vi "perform handshake.vi"(8 "error in":errorcluster, 9 "timeout":i32=-1, 11 "lvlibretls connection in":refnum<class "lvlibretls connection.lvclass">) -> (0 "error out":errorcluster, 3 "lvlibretls connection out":refnum<class "lvlibretls connection.lvclass">)   [LabVIEW 2016, in "lvlibretls connection.lvclass"]
doc: "tls_handshake() explicitly performs the TLS handshake. It is only necessary to call this function if you need to guarantee that the handshake has completed, as both tls_read() and tls_write() automatically perform the TLS handshake when necessary."
uses:
  lvlibretls connection.lvclass
  lvlibretls connection.lvclass/lvlibretls connection.ctl
  tls library paths.vi
  lv tls dll.lvlib
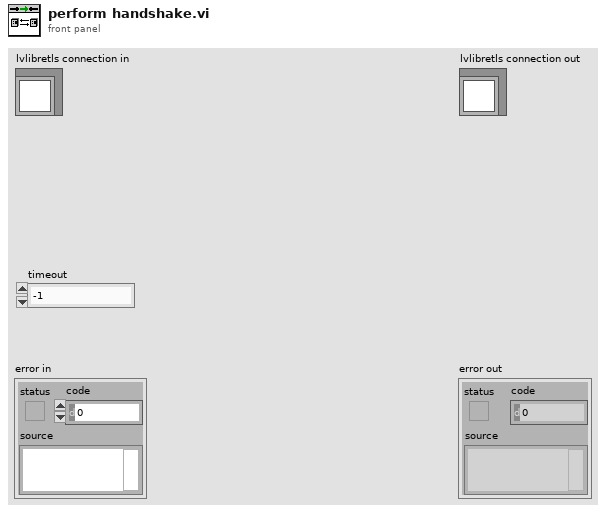
[diagram p1: front panel]
types:
  T1 = enum16{"Standard", "Buffered", "CRLF", "Immediate"}
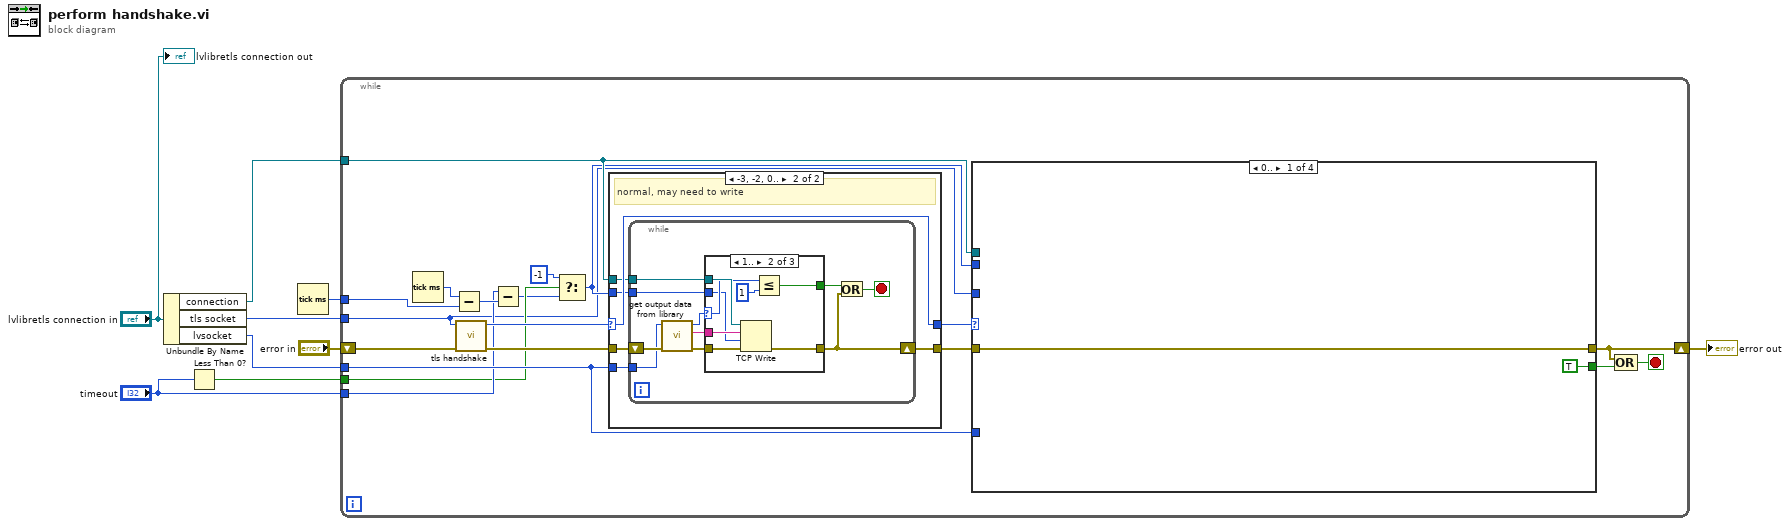
[diagram p0: block diagram]
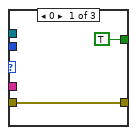
[diagram p3: hidden frame]
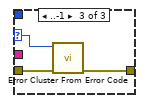
[diagram p4: hidden frame]
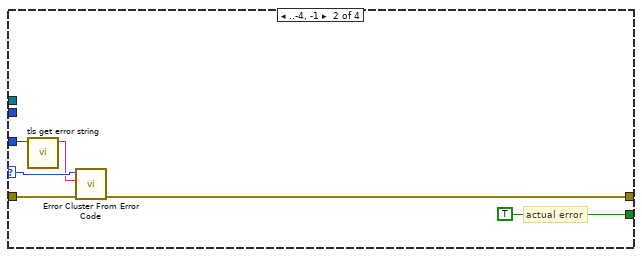
[diagram p5: hidden frame]
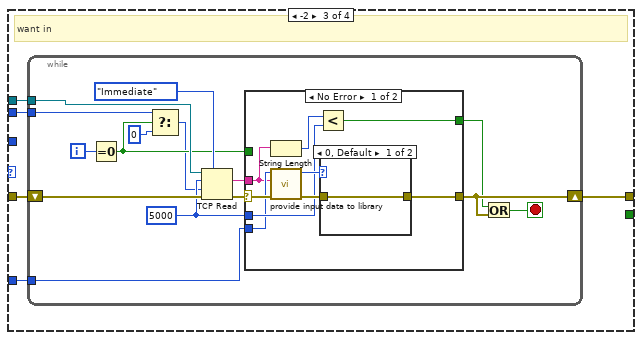
[diagram p6: hidden frame]
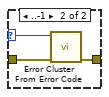
[diagram p7: hidden frame]
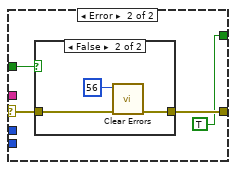
[diagram p8: hidden frame]
diagram:
  n1 = Unbundle By Name("lvlibretls connection in") -> ("connection"=w7:refnum<k5>, "tls socket"=w8:u64, "lvsocket"=w6:u64)
  n2 = Less Than 0?(x="timeout") -> (x < 0?=w2:bool)
  n3 = Tick Count (ms)() -> (millisecond timer value=w1:u32)
  n4 = while {
    shift-right: [w27] -> w4
    shift-left: "error in" -> [w28]
    tunnel: w8 -> [w10]
    tunnel: w7 -> [w19]
    tunnel: w6 -> [w20]
    tunnel: "timeout" -> [w15]
    tunnel: w2 -> [w14]
    tunnel: w1 -> [w17]
    stop <- w26 stop-if-true
    n5 = Tick Count (ms)() -> (millisecond timer value=w18:u32)
    n6 = Subtract(x=w18, y=w17) -> (x-y=w16:u32)
    n7 = call "tls handshake.vi"("error in"=w28, "tls context"=w10) -> ("error out"=w21:errorcluster, "return"=w24:i32)  [unwired: 8 in]
    n8 = Subtract(x=w15, y=w16) -> (x-y=w13:i32)
    n9 = Select(t=-1, s=w14, f=w13) -> (s? t:f=w11:i32)
    n10 = case shown="-3, -2, 0.." w24 {
      selector: w24 -> [w29 w36]
      tunnel: [w29 w36] -> w23
      tunnel: [w30 w34] -> w22
      tunnel: w21 -> [w30 w35]
      tunnel: w20 -> [_ w33]
      tunnel: w19 -> [_ w32]
      tunnel: w11 -> [_ w31]
      frame Default {
      }
      frame -3, -2, 0.. {
        # "normal, may need to write"
        n11 = while {
          shift-right: [w43] -> w34
          shift-left: w35 -> [w46]
          tunnel: w33 -> [w42]
          tunnel: w32 -> [w41]
          tunnel: w31 -> [w37]
          stop <- w40 stop-if-true
          n12 = call "get output data from library.vi"("error in"=w46, "lvsocket"=w42) -> ("error out"=w45:errorcluster, "data"=w38:string, "err"=w44:i32)  [unwired: 7 in]
          n13 = case shown="1.." w44 {
            selector: w44 -> [_ w52 w58]
            tunnel: w45 -> [w48 w56 w59]
            tunnel: [w48 w55 w57] -> w43
            tunnel: w38 -> [_ w54 _]
            tunnel: w41 -> [_ w53 _]
            tunnel: [TRUE w50 _] -> w39
            tunnel: w37 -> [_ w49 _]
            frame 0 {
            }
            frame 1.. {
              n14 = TCP Write(connection ID=w53, data in=w54, error in (no error)=w56, 9:w49) -> (error out=w55:errorcluster)  [unwired: 2 out]
              n15 = Less Or Equal?(x=w52, y=1) -> (x <= y?=w50:bool)
            }
            frame ..-1 {
              n16 = call <vilib>:"Error Cluster From Error Code.vi"("error in (no error)"=w59, "error code (0)"=w58) -> ("error out"=w57:errorcluster)  [unwired: 7 in]
            }
          }
          n17 = Or(x=w39, y=w43) -> (x .or. y?=w40:bool)
        }
      }
    }
    n18 = case shown="0.." w23 {
      selector: w23 -> [_ w67 _ _]
      tunnel: [w61 w66 w70 w109] -> w27
      tunnel: [TRUE TRUE _ _] -> w25
      tunnel: w19 -> [_ _ w72 _]
      tunnel: w20 -> [_ _ w71 _]
      tunnel: w22 -> [w61 w64 w69 w109]
      tunnel: w11 -> [_ _ w68 _]
      tunnel: w10 -> [_ w62 _ _]
      frame 0.. {
      }
      frame ..-4, -1 {
        # "actual error"
        n19 = call "tls get error string.vi"("tls context"=w62) -> ("error string"=w63:string)  [unwired: 9 in, 1 out]
        n20 = call <vilib>:"Error Cluster From Error Code.vi"("error in (no error)"=w64, "error message (\"\")"=w63, "error code (0)"=w67) -> ("error out"=w66:errorcluster)  [unwired: 6 in]
      }
      frame -2 {
        # "want in"
        n21 = while {
          tunnel: w72 -> [w87]
          tunnel: w71 -> [w84]
          shift-right: [w82] -> w70
          shift-left: w69 -> [w83]
          tunnel: w68 -> [w75]
          i -> [w81]
          stop <- w80 stop-if-true
          w78 = 5000 ("bytes to read")
          n22 = Equal To 0?(x=w81) -> (x = 0?=w76:bool)
          n23 = Select(t=w75, s=w76, f=0 ("timeout ms (25000)")) -> (s? t:f=w73:i32)
          n24 = TCP Read(connection ID=w87, bytes to read=w78, error in (no error)=w83, 7:T1."Immediate" ("mode (standard)"), 9:w73) -> (data out=w77:string, error out=w85:errorcluster)  [unwired: 1 out]
          n25 = case shown="No Error" w85 {
            selector: w85 -> [w96 w104]
            tunnel: w77 -> [w88 _]
            tunnel: w84 -> [w89 _]
            tunnel: [w93 w103] -> w82
            tunnel: w76 -> [_ w102]
            tunnel: [w90 TRUE] -> w79
            tunnel: w78 -> [w91 _]
            frame No Error {
              n26 = String Length(string=w88) -> (length=w92:i32)
              n27 = call "provide input data to library.vi"("error in"=w96, "data in"=w88, "lvsocket"=w89) -> ("error out"=w95:errorcluster, "return"=w94:i32)  [unwired: 7 in]
              n28 = Less?(x=w92, y=w91) -> (x < y?=w90:bool)
              n29 = case shown="0, Default" w94 {
                selector: w94 -> [_ w99]
                tunnel: w95 -> [w97 w100]
                tunnel: [w97 w98] -> w93
                frame 0, Default {
                }
                frame ..-1 {
                  n30 = call <vilib>:"Error Cluster From Error Code.vi"("error in (no error)"=w100, "error code (0)"=w99) -> ("error out"=w98:errorcluster)  [unwired: 7 in]
                }
              }
            }
            frame Error {
              n31 = case shown="False" w102 {
                tunnel: w104 -> [w105 w108]
                tunnel: [w105 w107] -> w103
                frame True {
                }
                frame False {
                  n32 = call <vilib>:"Clear Errors.vi"("error in (no error)"=w108, "specific error code to clear (0: all)"=56) -> ("error out"=w107:errorcluster)  [unwired: 4 in, 1 out]
                }
              }
            }
          }
          n33 = Or(x=w79, y=w82) -> (x .or. y?=w80:bool)
        }
      }
      frame -3 {
        # "want out"
      }
    }
    n34 = Compound Arithmetic op=OR(w27, w25) -> (w26:bool)
  }
  "error out" <- w4
  "lvlibretls connection out" <- "lvlibretls connection in"
